vi "set_Manufacturer.vi"(8 "error in (no error)":errorcluster, 10 "Manufacturer":string, 11 "GenericDetector in":refnum<class "GenericDetector.lvclass">) -> (0 "error out":errorcluster, 3 "GenericDetector out":refnum<class "GenericDetector.lvclass">)   [LabVIEW 2010, in "GenericDetector.lvclass"]
uses:
  GenericDetector.lvclass
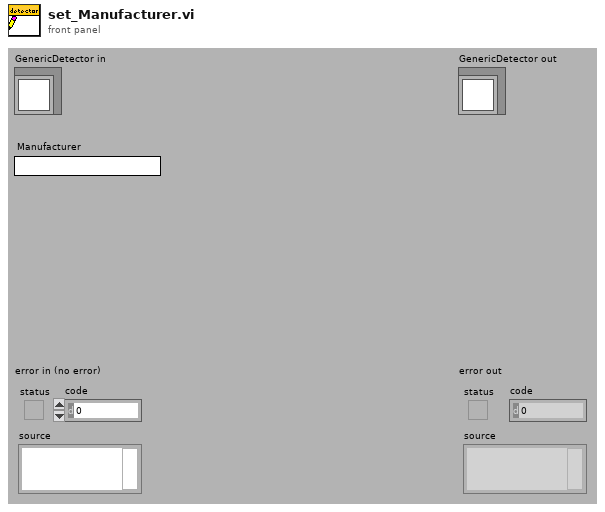
[diagram p1: front panel]
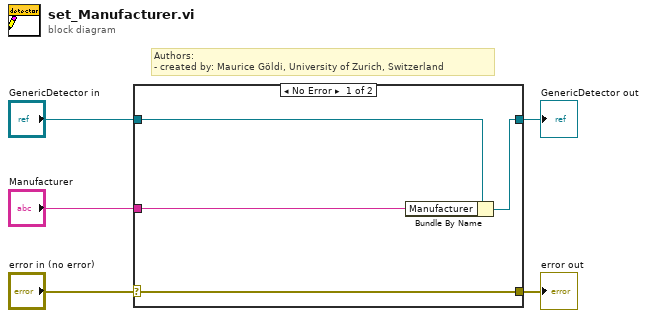
[diagram p0: block diagram]
diagram:
  # "Authors: \n- created by: Maurice Göldi, University of Zurich, Switzerland"
  n1 = case shown="No Error" "error in (no error)" {
    selector: "error in (no error)" -> [w9 w10]
    tunnel: [w9 w10] -> w4
    tunnel: [w7 w11] -> w2
    tunnel: "GenericDetector in" -> [w8 w11]
    tunnel: "Manufacturer" -> [w6 _]
    frame No Error {
      n2 = Bundle By Name(cluster=w8, "Manufacturer"=w6) -> (w7:refnum<class "GenericDetector.lvclass">)
    }
    frame Error {
    }
  }
  "error out" <- w4
  "GenericDetector out" <- w2
